vi "Launch Logger.vi"(8 "error in":errorcluster, 9 "Log Level":T1, 10 "Log Option":T2, 11 "Logger Manager":refnum<data-value>) -> (0 "error out":errorcluster, 3 "Logger Manager Out":refnum<data-value>)   [LabVIEW 2020]
uses:
  Logger Manager/Logger Manager.lvclass
  <vilib>/ActorFramework/Actor/Actor.lvclass
  File Logger/File Logger.lvclass
  Generic Logger/Generic Logger.lvclass
  Console Logger/Console Logger.lvclass
  C:/Program Files (x86)/National Instruments/LabVIEW 2020/vi.lib/ActorFramework/Actor/Actor.lvclass
  E:/NI I Program/Actor FCT Frame/Logging/Generic Logger/Generic Logger.lvclass
  Define/Log Option.ctl
  Logging.lvlib
  Define/Log Level.ctl
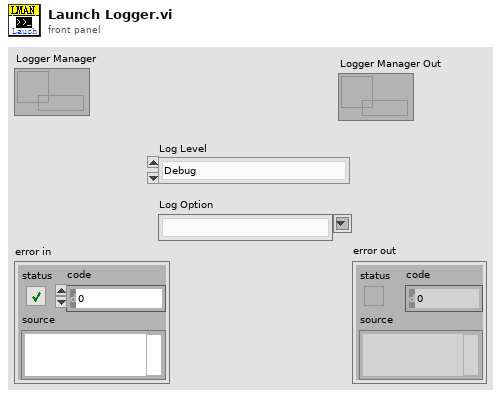
[diagram p1: front panel]
types:
  T1 = typedef "Logging.lvlib/Log Level.ctl" = enum16{"Debug", "Info", "Warn", "Error"}
  T2 = typedef "Logging.lvlib/Log Option.ctl" = string
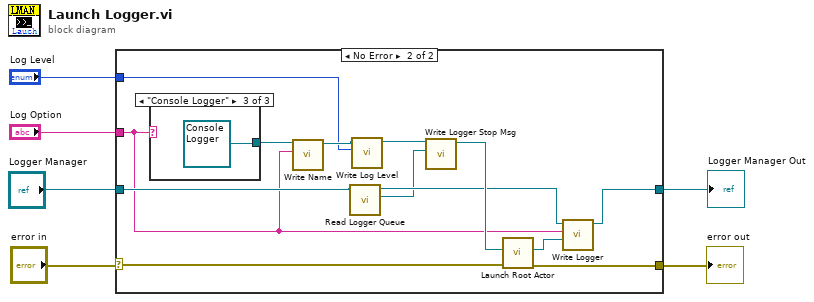
[diagram p0: block diagram]
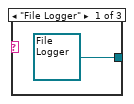
[diagram p3: hidden frame]
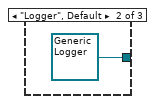
[diagram p4: hidden frame]
diagram:
  n1 = case shown="No Error" "error in" {
    selector: "error in" -> [w7 w15]
    tunnel: "Logger Manager" -> [w8 w12]
    tunnel: "Log Option" -> [_ w9]
    tunnel: [w8 w20] -> w6
    tunnel: "Log Level" -> [_ w17]
    tunnel: [w7 w16] -> w3
    frame Error {
    }
    frame No Error {
      n2 = case shown="\"Console Logger\"" w9 {
        tunnel: [refnum<class "File Logger.lvclass"> refnum ("Logger.lvlib:File Logger.lvclass") refnum<class "Generic Logger.lvclass"> refnum ("Logger.lvlib:Logger.lvclass") refnum<class "Console Logger.lvclass"> refnum ("Logger.lvlib:Console Logger.lvclass")] -> w19
        frame "File Logger" {
        }
        frame "Logger", Default {
        }
        frame "Console Logger" {
        }
      }
      n3 = call-dynamic "Write Name.vi"("Name"=w9, "Logger in"=w19) -> ("Logger out"=w18:refnum<class "Generic Logger.lvclass">)  [unwired: 8 in, 1 out]
      n4 = call "Read Logger Queue.vi"("Logger Manager In"=w12) -> ("Logger Stop Msg"=w10:refnum<queue>, "Logger Manager Out"=w11:refnum<data-value>)  [unwired: 8 in, 1 out]
      n5 = call-dynamic "Write Log Level.vi"("Log Level"=w17, "Logger in"=w18) -> ("Logger out"=w14:refnum<class "Generic Logger.lvclass">)  [unwired: 8 in, 1 out]
      n6 = call "Write Logger Stop Msg.vi"("Logger Stop Msg"=w10, "Logger in"=w14) -> ("Logger out"=w13:refnum<class "Generic Logger.lvclass">)  [unwired: 8 in, 1 out]
      n7 = call <vilib>:"Launch Root Actor.vi"("error in (no error)"=w15, "Actor"=w13) -> ("error out"=w16:errorcluster, "Actor's Enqueuer"=w21:refnum<class "Message Enqueuer.lvclass">)  [unwired: 8 in]
      n8 = call "Write Logger.vi"("Logger"=w21, "Name"=w9, "Logger Manager In"=w11) -> ("Logger Manager Out"=w20:refnum<data-value>)  [unwired: 7 in, 1 out]
    }
  }
  "error out" <- w3
  "Logger Manager Out" <- w6
